vi "WLAN_FrameSync.vi"(11 "input cluster":cluster{"t0":dbl, "dt":dbl, "Y":cdb[]}) -> (2 "is valid packet?":bool, 3 "output cluster":cluster{"t0":dbl, "dt":dbl, "Y":cdb[]})   [LabVIEW 2014]
uses:
  <vilib>/Analysis/2dsp.llb/1D Cross Correlation (CDB).vi
  <vilib>/Analysis/NI_AALPro.lvlib
panel:
  out "x > y?":bool
  out "Waveform Graph 5":dbl[](graph)
  out "Waveform Graph 4":dbl[][](graph)
  out "Waveform Graph 3":dbl[][](graph)
  out "x-y":i32
  out "Waveform Graph 2":dbl[](graph)
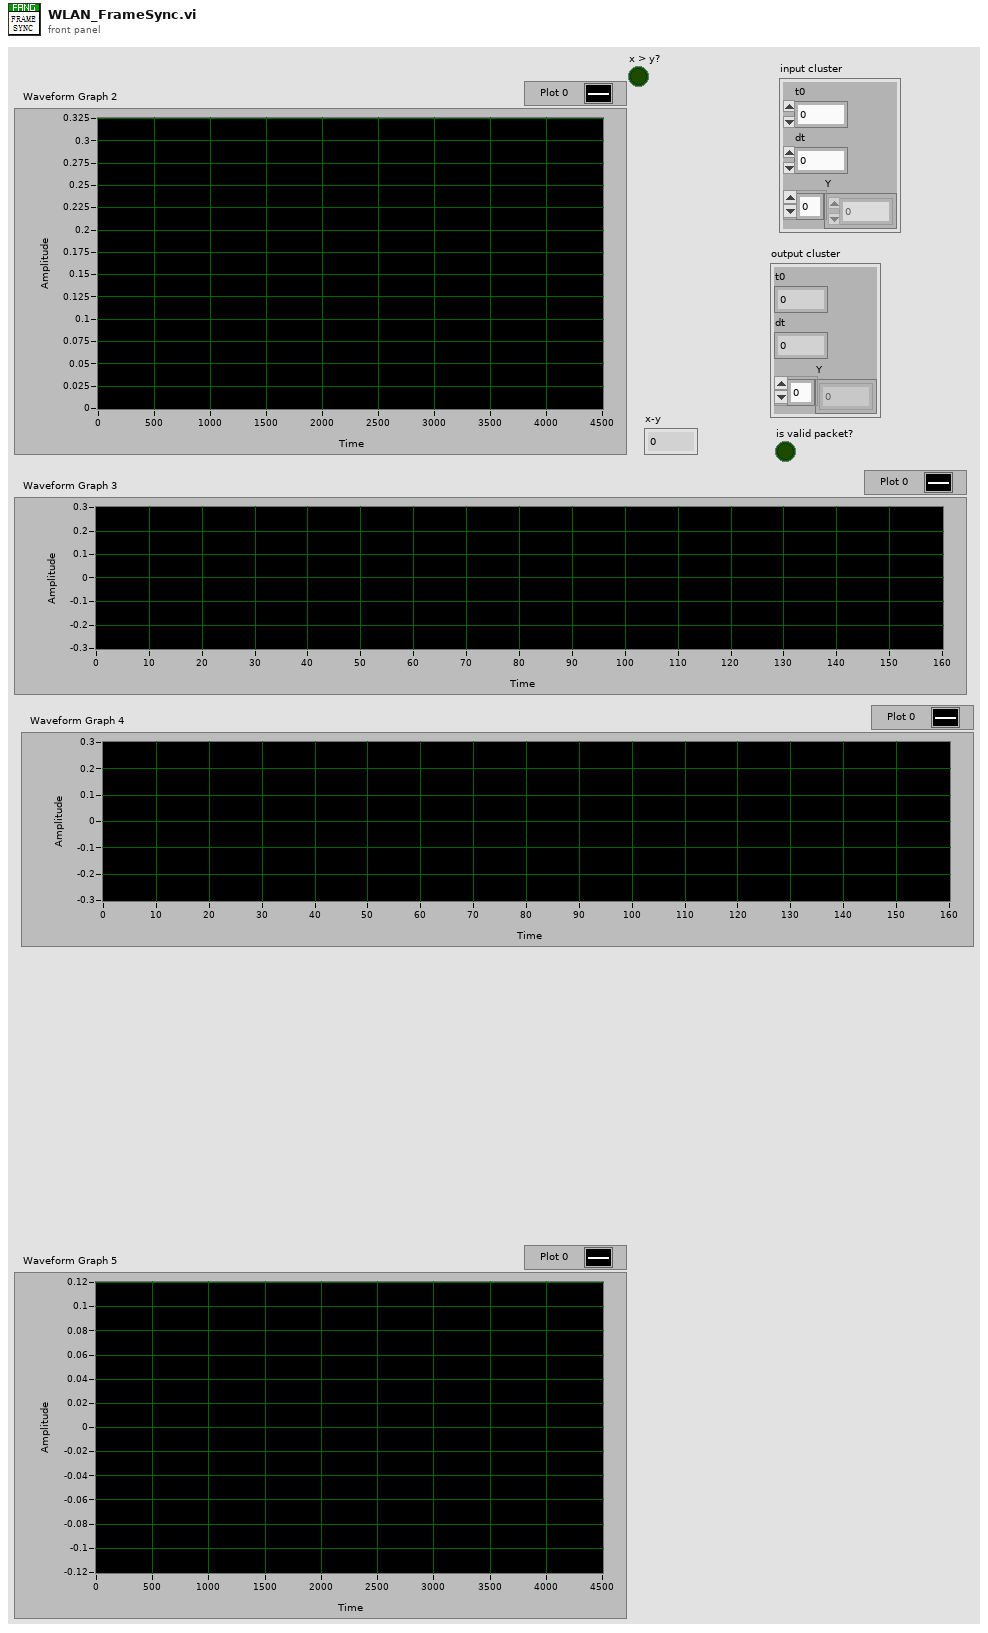
[diagram p1: front panel]
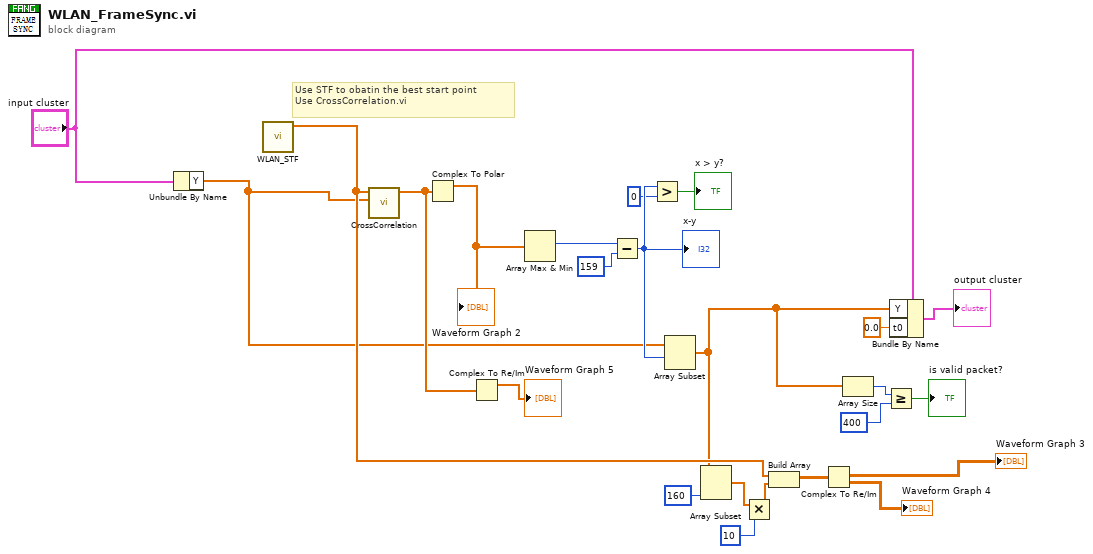
[diagram p0: block diagram]
diagram:
  # "Use STF to obatin the best start point\nUse CrossCorrelation.vi"
  n1 = Unbundle By Name("input cluster") -> ("Y"=w1:cdb[])
  n2 = call "WLAN_STF.vi"() -> ("STF"=w17:cdb[])  [unwired: 11 in]
  n3 = call-poly <vilib>:"CrossCorrelation.vi"("Y"=w1, "X"=w17) -> ("Rxy"=w6:cdb[])  [unwired: 8 in, 1 out]
  n4 = Complex To Polar(r * e^(i*theta)=w6) -> (r=w24:dbl[])  [unwired: 1 out]
  "Waveform Graph 2" <- w24
  n5 = Complex To Re/Im(x + iy=w6) -> (x=→"Waveform Graph 5":dbl[])  [unwired: 1 out]
  n6 = Array Max & Min(array=w24) -> (max index (indices)=w22:i32)  [unwired: 3 out]
  n7 = Subtract(x=w22, y=159) -> (x-y=w4:i32)
  "x-y" <- w4
  n8 = Greater?(x=w4, y=0) -> (0:→"x > y?":bool)
  n9 = Array Subset(array=w1, index=w4) -> (w7:cdb[])  [unwired: 1 in]
  n10 = Array Subset(array=w7, length=160) -> (w16:cdb[])  [unwired: 1 in]
  n11 = Multiply(x=w16, y=10 ("length")) -> (x*y=w14:cdb[])
  n12 = Build Array(w17, w14) -> (w13:cdb[][])
  n13 = Complex To Re/Im(x + iy=w13) -> (x=→"Waveform Graph 3":dbl[][], y=→"Waveform Graph 4":dbl[][])
  n14 = Array Size(array=w7) -> (size(s)=w10:i32)
  n15 = Greater Or Equal?(x=w10, y=400) -> (x >= y?=→"is valid packet?":bool)
  n16 = Bundle By Name(cluster="input cluster", "Y"=w7, "t0"=0.0) -> (→"output cluster":cluster{"t0":dbl, "dt":dbl, "Y":cdb[]})
